vi "CheckForError.vi"(8 "Error In":errorcluster) -> (0 "error out":errorcluster)   [LabVIEW 2018, in "ErrorHandler.lvlib"]
uses:
  ErrorHandler.lvlib
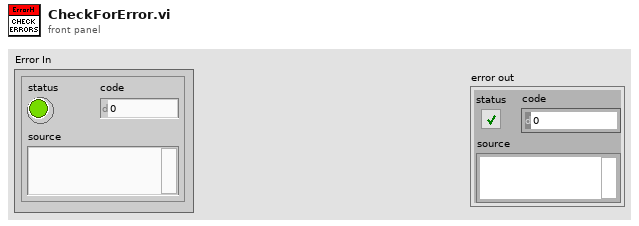
[diagram p1: front panel]
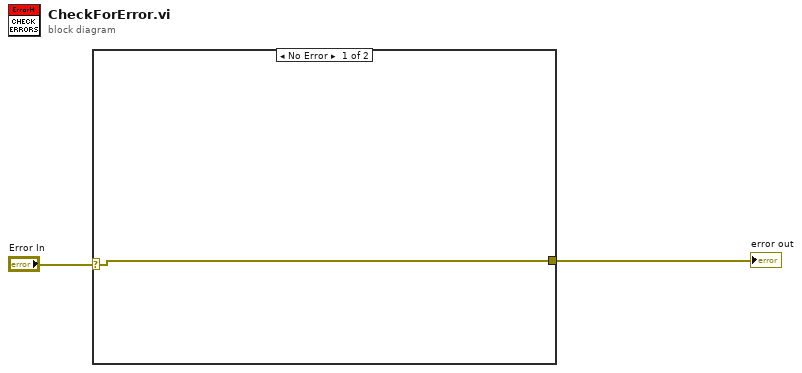
[diagram p0: block diagram]
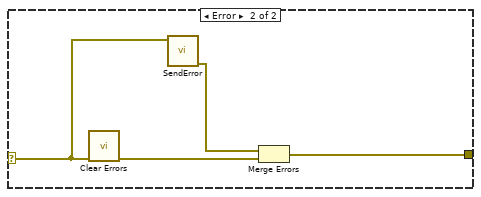
[diagram p2: hidden frame]
diagram:
  n1 = case shown="No Error" "Error In" {
    selector: "Error In" -> [w3 w7]
    tunnel: [w3 w5] -> w2
    frame No Error {
    }
    frame Error {
      n2 = call <vilib>:"Clear Errors.vi"("error in (no error)"=w7) -> ("error out"=w6:errorcluster)  [unwired: 5 in, 1 out]
      n3 = call "SendError.vi"("Payload"=w7) -> ("error out"=w4:errorcluster)  [unwired: 9 in, 1 out]
      n4 = Merge Errors(w4, w6) -> (w5:errorcluster)
    }
  }
  "error out" <- w2
